vi "EVENODDSIGNINFO.vi"(1 "Numeric":dbl) -> (0 "concatenated string":string)   [LabVIEW 2019]
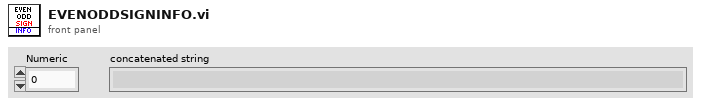
[diagram p1: front panel]
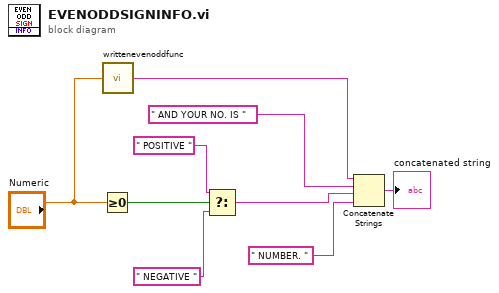
[diagram p0: block diagram]
diagram:
  n1 = Greater Or Equal To 0?(x="Numeric") -> (x >= 0?=w1:bool)
  n2 = call "writtenevenoddfunc.vi"("Numeric"="Numeric") -> ("concatenated string"=w5:string)
  n3 = Select(t=" POSITIVE ", s=w1, f=" NEGATIVE ") -> (s? t:f=w7:string)
  n4 = Concatenate Strings(w5, " AND YOUR NO. IS " ("string"), w7, " NUMBER. " ("string")) -> (→"concatenated string":string)
